vi "Startup.vi"(6 "LabVIEW Web Service":refnum<class "Web Service.lvclass">) -> ()   [LabVIEW 2019]
uses:
  <vilib>/wsapi/Web Service.lvclass
  Configuration/Global_Configurations.vi
panel:
  # "Use the web service input terminal to call the VIs on the Service subpalette of the Web Services palette. Do not remove it from the connector pane unless you don't need access to the palette."
  # "Any additional terminals added to the connector pane of a startup VI will be ignored."
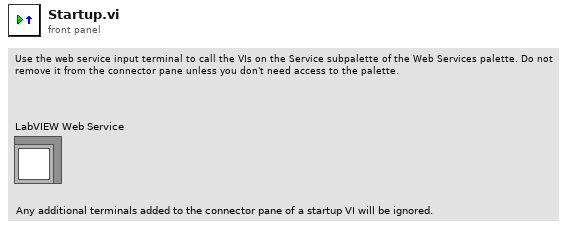
[diagram p1: front panel]
types:
  T1 = cluster{"Path":path, "Name":string, "Authors":string, "Keywords":string, "Description":string, "Cameras":cluster{"Base URL":string, "Path":string, "Name":string}[], "Sampling":cluster{"Sampled Variable":string, "Delta":dbl}[], "Sampling Freq":u32}[]
  T2 = cluster{"Path":path, "Name":string, "Authors":string, "Keywords":string, "Description":string, "Cameras":cluster{"Base URL":string, "Path":string, "Name":string}[], "Sampling":cluster{"Sampled Variable":string, "Delta":dbl}[], "Sampling Freq":u32}
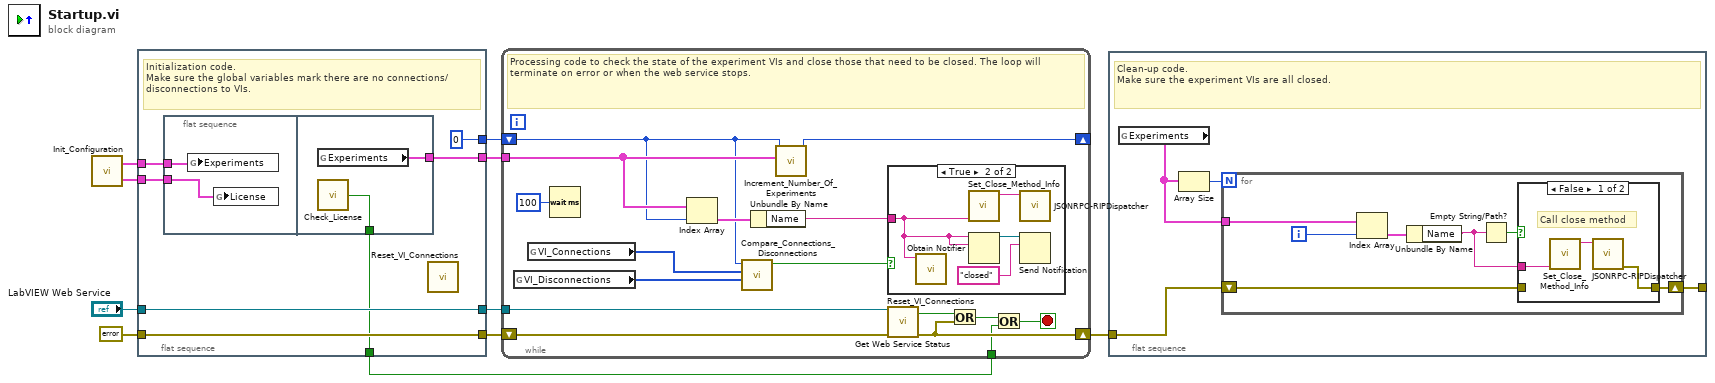
[diagram p0: block diagram]
diagram:
  n1 = call "Init_Configuration.vi"() -> ("License"=w1:cluster{"ID":string, "Number":string}, "Experiments"=w3:T1)  [unwired: 2 in]
  n2 = flat-sequence {
    tunnel: "LabVIEW Web Service" -> [w17]
    tunnel: [w17] -> w9
    tunnel: [w16] -> w8
    tunnel: errorcluster {"status"=FALSE, "code"=0, "source"=""} ("error constant") -> [w16]
    tunnel: [0] -> w5
    tunnel: [w14] -> w4
    tunnel: w3 -> [w13]
    tunnel: [w12] -> w2
    tunnel: w1 -> [w11]
    frame #0 {
      # "Initialization code.\nMake sure the global variables mark there are no connections/disconnections to VIs."
      n3 = flat-sequence {
        tunnel: w13 -> [w19]
        tunnel: w11 -> [w18]
        tunnel: [w21] -> w14
        tunnel: [w20] -> w12
        frame #0 {
          n4 = global write "Global_Configurations.vi" "Experiments"(w19) -> ()
          n5 = global write "Global_Configurations.vi" "License"(w18) -> ()
        }
        frame #1 {
          n6 = global read "Global_Configurations.vi" "Experiments"() -> (w21:T1)
          n7 = call "Check_License.vi"() -> ("Boolean"=w20:bool)  [unwired: 2 in]
        }
      }
      n8 = call "Reset_VI_Connections.vi"() -> ()  [unwired: 12 in]
    }
  }
  n9 = while {
    tunnel: w9 -> [w36]
    shift-right: [w34] -> w6
    shift-left: w8 -> [w35]
    shift-right: [w31] -> _
    shift-left: w5 -> [w25]
    tunnel: w4 -> [w26]
    tunnel: w2 -> [w22]
    stop <- w24 stop-if-true
    # "Processing code to check the state of the experiment VIs and close those that need to be closed. The loop will terminate on error or when the web service stops."
    n10 = global read "Global_Configurations.vi" "VI_Disconnections"() -> (w28:u8[])
    n11 = global read "Global_Configurations.vi" "VI_Connections"() -> (w29:u8[])
    n12 = Wait (ms)(milliseconds to wait=u32 100) -> ()  [unwired: 1 out]
    n13 = Index Array(array=w26, index=w25) -> (element=w32:T2)
    n14 = call "Compare_Connections_Disconnections.vi"("VI_Disconnections"=w28, "VI_Connections"=w29, "Numeric"=w25) -> ("Boolean"=w27:bool)  [unwired: 8 in]
    n15 = Unbundle By Name(w32) -> ("Name"=w30:string)
    n16 = call "Increment_Number_Of_Experiments.vi"("Experiments"=w26, "Numeric"=w25) -> ("f"=w31:i32)  [unwired: 9 in]
    n17 = case shown="True" w27 {
      tunnel: w30 -> [_ w38]
      frame False {
      }
      frame True {
        n18 = call "Reset_VI_Connections.vi"("expId"=w38) -> ()  [unwired: 11 in]
        n19 = call "Set_Close_Method_Info.vi"("expId"=w38) -> ("String"=w41:string)  [unwired: 10 in]
        n20 = Obtain Notifier(name (unnamed)=w38, notification data type=w38) -> (notifier out=w40:refnum<notifier>)  [unwired: 2 in, 2 out]
        n21 = call "JSONRPC-RIPDispatcher.vi"("input string"=w41) -> ()  [unwired: 9 in, 2 out]
        n22 = Send Notification(notification="closed", notifier=w40) -> ()  [unwired: 1 in, 2 out]
      }
    }
    n23 = call <vilib>:"Get Web Service Status.vi"("LabVIEW Web Service"=w36, "error in (no error)"=w35) -> ("service stopping?"=w37:bool, "error out"=w34:errorcluster)  [unwired: 11 in, 1 out]
    n24 = Or(x=w37, y=w34) -> (x .or. y?=w23:bool)
    n25 = Or(x=w23, y=w22) -> (x .or. y?=w24:bool)
  }
  n26 = flat-sequence {
    tunnel: w6 -> [w44]
    tunnel: [w43] -> _
    frame #0 {
      # "Clean-up code.\nMake sure the experiment VIs are all closed."
      n27 = global read "Global_Configurations.vi" "Experiments"() -> (w42:T1)
      n28 = Array Size(array=w42) -> (size(s)=w45:i32)
      n29 = for {
        N: w45 -> [_]
        shift-right: [w48] -> w43
        shift-left: w44 -> [w47]
        tunnel: w42 -> [w46]
        i -> [w51]
        n30 = Index Array(array=w46, index=w51) -> (element=w52:T2)
        n31 = Unbundle By Name(w52) -> ("Name"=w49:string)
        n32 = Empty String/Path?(string/path=w49) -> (empty?=w50:bool)
        n33 = case shown="False" w50 {
          tunnel: w49 -> [w54 _]
          tunnel: [w53 w56] -> w48
          tunnel: w47 -> [_ w56]
          frame False {
            # "Call close method"
            n34 = call "Set_Close_Method_Info.vi"("expId"=w54) -> ("String"=w55:string)  [unwired: 10 in]
            n35 = call "JSONRPC-RIPDispatcher.vi"("input string"=w55) -> ("error out"=w53:errorcluster)  [unwired: 9 in, 1 out]
          }
          frame True {
          }
        }
      }
    }
  }
